vi "TMCM351-SetAnalogueVoltage.vi"(4 "错误输入":errorcluster caption="错误输入（无错误）", 5 "数据":enum16{"3.3v", "10v"}(ring), 7 "com in":refnum<visa-resource-name>) -> (0 "错误输出":errorcluster, 1 "ReadOut":i32, 3 "com out":refnum<visa-resource-name>)   [LabVIEW 2018]
uses:
  module_param.vi
panel:
  out "return out":u8[](array[numeric])
  out "添加的数组":u8[](array[numeric]) format="%x"
  # "读取IO口"
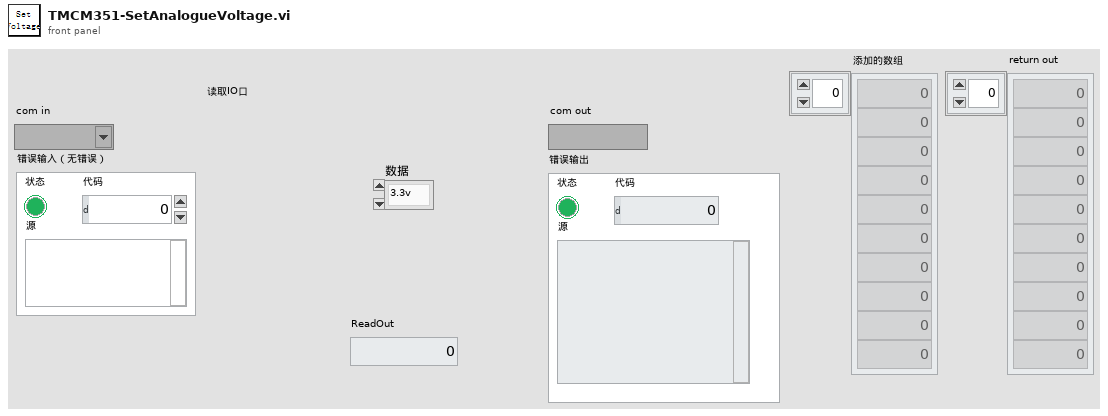
[diagram p1: front panel]
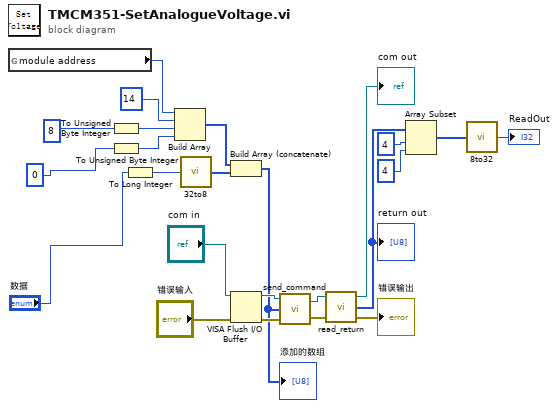
[diagram p0: block diagram]
diagram:
  n1 = global read "module_param.vi" "module address"() -> (w10:u8)
  n2 = To Unsigned Byte Integer(number=u8 8 ("数字")) -> (unsigned 8bit integer=w11:u8)
  n3 = To Unsigned Byte Integer(number=0) -> (unsigned 8bit integer=w9:u8)
  n4 = To Long Integer(number="数据") -> (32bit integer=w17:i32)
  n5 = Build Array(w10, u8 14, w11, w9) -> (w19:u8[])
  n6 = call "32to8.vi"("32data_in"=w17) -> ("8Array"=w16:u8[])
  n7 = Build Array (concatenate)(w19, w16) -> (w18:u8[])
  "添加的数组" <- w18
  n8 = VISA Flush I/O Buffer(VISA resource name="com in", error in (no error)="错误输入") -> (VISA resource name out=w21:refnum<visa-resource-name>, error out=w20:errorcluster)  [unwired: 1 in]
  n9 = call "send_command.vi"("错误输入"=w20, 3:w18, "com in"=w21) -> ("错误输出"=w12:errorcluster, "com out"=w13:refnum<visa-resource-name>)
  n10 = call "read_return.vi"("错误输入（无错误）"=w12, "com in"=w13) -> ("错误输出"=→"错误输出":errorcluster, "return out"=w8:u8[], "com out"=→"com out":refnum<visa-resource-name>)  [unwired: 1 in]
  "return out" <- w8
  n11 = Array Subset(array=w8, index=4 ("索引"), length=4 ("长度")) -> (w5:u8[])
  n12 = call "8to32.vi"("Arrayin"=w5) -> ("data32"=→"ReadOut":i32)
